vi "读取表格多个sheet全部数据并分类.vi"(7 "错误 in":errorcluster caption="错误常量", 8 "各sheet名称数组":string[](array[string]), 10 "Cpk计算数量":i32, 11 "File in":path) -> (3 "存储数据 2":T1)   [LabVIEW 2014]
uses:
  Controls/SelectCamLight.ctl
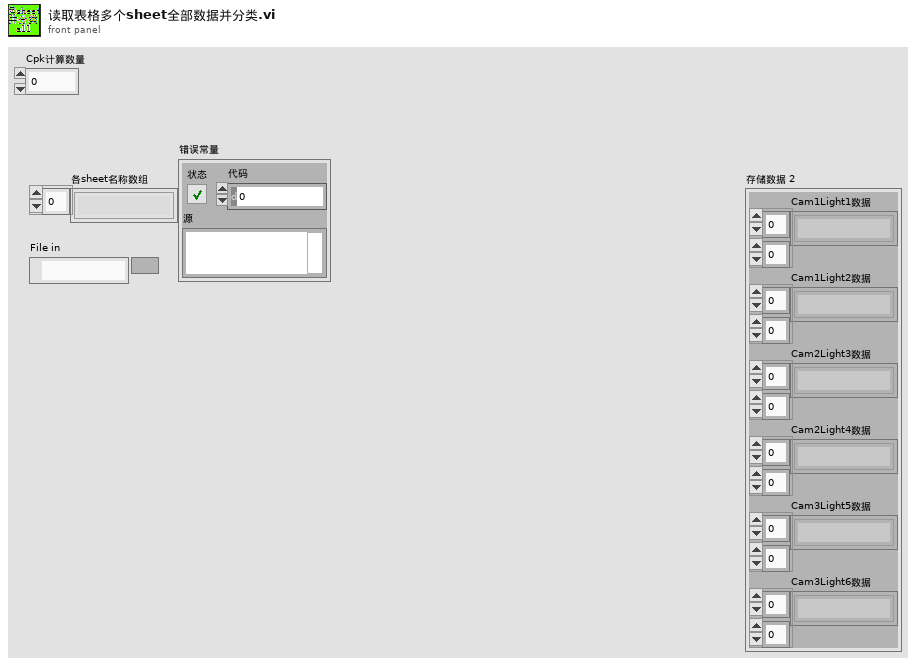
[diagram p1: front panel]
types:
  T1 = cluster{"Cam1Light1数据":string[][], "Cam1Light2数据":string[][], "Cam2Light3数据":string[][], "Cam2Light4数据":string[][], "Cam3Light5数据":string[][], "Cam3Light6数据":string[][]}
  T2 = enum16{"打开表格", "新增sheet", "读取sheet指定位置数据", "读取sheet整个数据", "写入sheet整个数据", "数据存到本机", "关闭表格"}
  T3 = typedef "SelectCamLight.ctl" = enum16{"相机1光源1", "相机1光源2", "相机2光源3", "相机2光源4", "相机3光源5", "相机3光源6"}
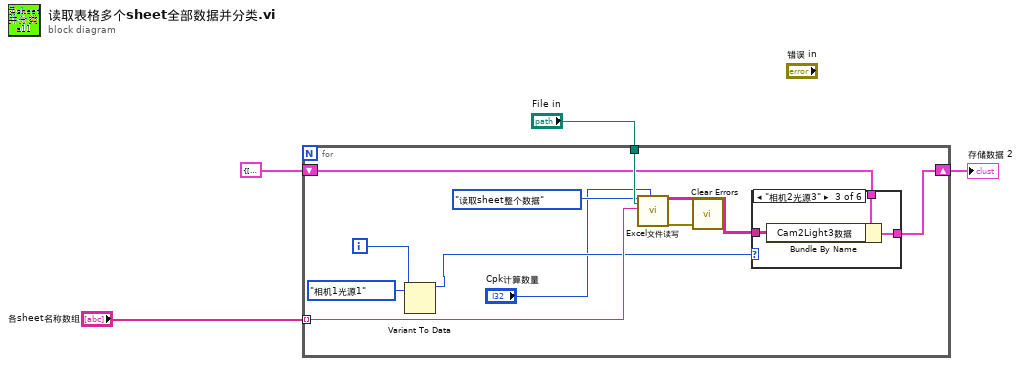
[diagram p0: block diagram]
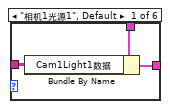
[diagram p2: hidden frame]
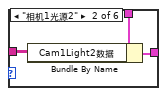
[diagram p3: hidden frame]
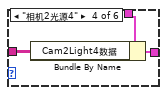
[diagram p4: hidden frame]
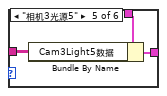
[diagram p5: hidden frame]
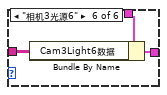
[diagram p6: hidden frame]
diagram:
  n1 = for {
    tunnel: "File in" -> [w14]
    tunnel: "各sheet名称数组" -> [w13] mode=indexing
    shift-right: [w10] -> w4
    shift-left: T1 {"Cam1Light1数据"=[], "Cam1Light2数据"=[], "Cam2Light3数据"=[], "Cam2Light4数据"=[], "Cam3Light5数据"=[], "Cam3Light6数据"=[]} ("存储数据 2") -> [w11]
    i -> [w15]
    n2 = Variant To Data(type=SelectCamLight."相机1光源1" ("相机光源选项"), Variant=w15) -> (data=w12:T3)  [unwired: 1 in, 1 out]
    n3 = call "Excel文件读写.vi"("选项"=T2."读取sheet整个数据", "Path"=w14, "worksheet name"=w13, "Cpk计算数量"="Cpk计算数量") -> ("data"=w9:string[][], "error out"=w8:errorcluster)  [unwired: 14 in]
    n4 = call <vilib>:"Clear Errors.vi"("error in (no error)"=w8) -> ()  [unwired: 5 in, 2 out]
    n5 = case shown="\"相机2光源3\"" w12 {
      tunnel: w11 -> [w18 w21 w24 w27 w30 w33]
      tunnel: [w17 w20 w23 w26 w29 w32] -> w10
      tunnel: w9 -> [w16 w19 w22 w25 w28 w31]
      frame "相机1光源1", Default {
        n6 = Bundle By Name(cluster=w18, "Cam1Light1数据"=w16) -> (w17:T1)
      }
      frame "相机1光源2" {
        n7 = Bundle By Name(cluster=w21, "Cam1Light2数据"=w19) -> (w20:T1)
      }
      frame "相机2光源3" {
        n8 = Bundle By Name(cluster=w24, "Cam2Light3数据"=w22) -> (w23:T1)
      }
      frame "相机2光源4" {
        n9 = Bundle By Name(cluster=w27, "Cam2Light4数据"=w25) -> (w26:T1)
      }
      frame "相机3光源5" {
        n10 = Bundle By Name(cluster=w30, "Cam3Light5数据"=w28) -> (w29:T1)
      }
      frame "相机3光源6" {
        n11 = Bundle By Name(cluster=w33, "Cam3Light6数据"=w31) -> (w32:T1)
      }
    }
  }
  "存储数据 2" <- w4
